vi "script_target_dsf_configuration.vi"(5 "Plugin Timing":T3={"priority"=100, "decimation"=1, "offset"=0}, 7 "configuration version":cluster{"major":u32, "minor":u32, "fix":u32}={"major"=1, "minor"=0, "fix"=0}, 8 "error in":errorcluster, 9 "Target Threads":T1[](array[typedef]), 10 "Target Configuration":T7, 11 "vsd reference":refnum<k24>) -> (0 "error out":errorcluster)   [LabVIEW 2020]
uses:
  NationalInstruments.VeriStand.SystemDefinitionAPI
  controls/target_configuration_cluster.ctl
  <vilib>/addons/VeriStand Custom Device Scripting APIs/Data Sharing Framework/DSF Core.lvlibp/Typedefs/DSF Timing Info.ctl
  controls/thread_configuration_data.ctl
  controls/tx_transfer_group_configuration_data.ctl
  controls/tx_configuration_data.ctl
  controls/rx_transfer_group_configuration_data.ctl
  controls/rx_configuration_data.ctl
  <vilib>/addons/VeriStand Custom Device Scripting APIs/Data Sharing Framework/DSF Core.lvlibp/Typedefs/DSF Engine Plugin Configuration.ctl
  <vilib>/addons/VeriStand Custom Device Scripting APIs/Data Sharing Framework/DSF Core.lvlibp/Typedefs/Core Plugin Configuration.ctl
  <vilib>/addons/VeriStand Custom Device Scripting APIs/Data Sharing Framework/DSF Core.lvlibp/Typedefs/DSF Settings Info.ctl
  <vilib>/addons/VeriStand Custom Device Scripting APIs/Data Sharing Framework/DSF Core.lvlibp/Typedefs/DSF Engine Plugin Thread Configuration.ctl
  <vilib>/addons/VeriStand Custom Device Scripting APIs/Data Sharing Framework/DSF Core.lvlibp/Typedefs/Core Thread Configuration.ctl
  <vilib>/addons/VeriStand Custom Device Scripting APIs/Data Sharing Framework/DSF Core.lvlibp/Typedefs/DSF Engine Transfer Group Configuration.ctl
  <vilib>/addons/VeriStand Custom Device Scripting APIs/Data Sharing Framework/DSF Core.lvlibp/Typedefs/Core Group Configuration.ctl
  <vilib>/addons/VeriStand Custom Device Scripting APIs/Data Sharing Framework/DSF Core.lvlibp/Typedefs/DSF Direction.ctl
  <vilib>/addons/VeriStand Custom Device Scripting APIs/Data Sharing Framework/DSF Core.lvlibp/Typedefs/DSF Timeout Behavior.ctl
  <vilib>/addons/VeriStand Custom Device Scripting APIs/Data Sharing Framework/DSF Core.lvlibp/Typedefs/DSF Engine Transfer Configuration.ctl
  <vilib>/addons/VeriStand Custom Device Scripting APIs/Data Sharing Framework/DSF Core.lvlibp/Typedefs/Core Transfer Configuration.ctl
  <vilib>/addons/VeriStand Custom Device Scripting APIs/Data Sharing Framework/DSF Core.lvlibp/Typedefs/DSF Engine Channel Configuration.ctl
  <vilib>/addons/VeriStand Custom Device Scripting APIs/Data Sharing Framework/DSF Core.lvlibp/Typedefs/Core Channel Configuration.ctl
  <vilib>/addons/VeriStand Custom Device Scripting APIs/Data Sharing Framework/DSF Core.lvlibp/Typedefs/DSF Data Type.ctl
  <vilib>/addons/VeriStand Custom Device Scripting APIs/Data Sharing Framework/DSF Core.lvlibp/Typedefs/DSF Engine Framework Configuration.ctl
  <vilib>/addons/VeriStand Custom Device Scripting APIs/Data Sharing Framework/Data Sharing Framework Custom Device Scripting.lvlib
  <vilib>/addons/VeriStand Custom Device Scripting APIs/Data Sharing Framework/DSF Core.lvlibp
  <vilib>/addons/VeriStand Custom Device Scripting APIs/Data Sharing Framework/DSF Core.lvlibp/Classes/Configuration/Core/Plugin/Plugin Configuration.lvclass
  <vilib>/addons/VeriStand Custom Device Scripting APIs/Data Sharing Framework/DSF Core.lvlibp/Classes/Configuration/Core/Thread/Thread Configuration.lvclass
  <vilib>/addons/VeriStand Custom Device Scripting APIs/Data Sharing Framework/DSF Core.lvlibp/Classes/Configuration/Core/Group/Group Configuration.lvclass
  <vilib>/addons/VeriStand Custom Device Scripting APIs/Data Sharing Framework/DSF Core.lvlibp/Classes/Configuration/Core/Transfer/Transfer Configuration.lvclass
  <vilib>/addons/VeriStand Custom Device Scripting APIs/Data Sharing Framework/DSF Core.lvlibp/Classes/Configuration/Core/Channel/Channel Configuration.lvclass
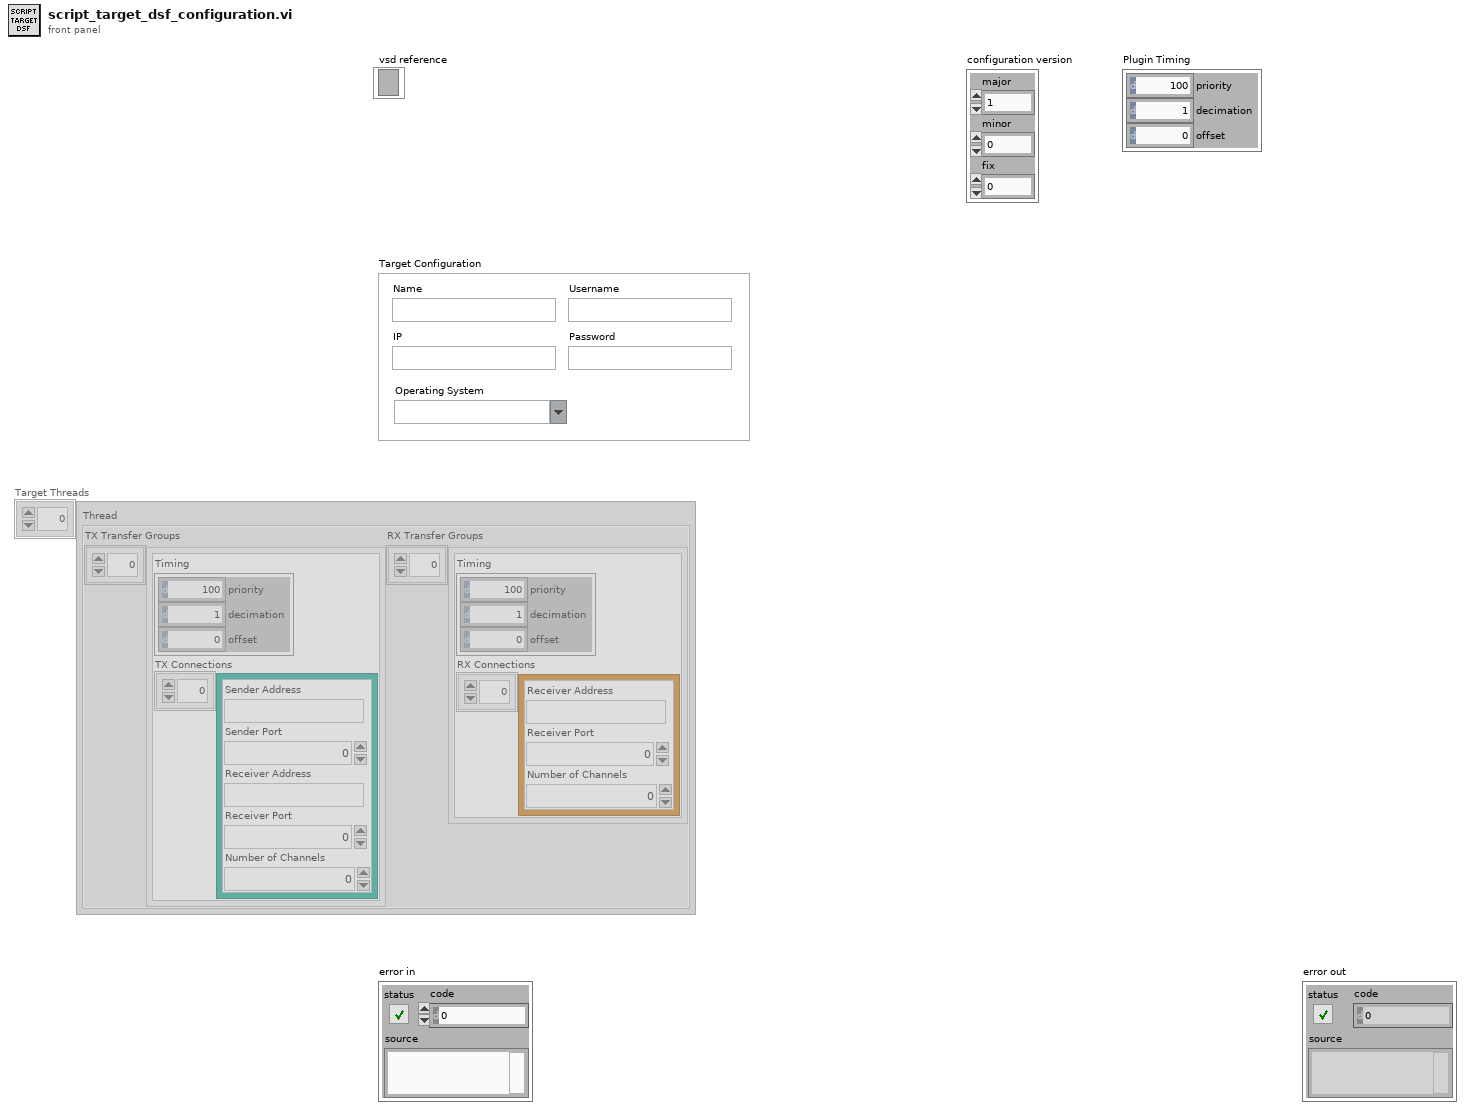
[diagram p1: front panel]
types:
  T1 = typedef "thread_configuration_data.ctl" = cluster{"TX Transfer Groups":T2[], "RX Transfer Groups":T5[]}
  T2 = typedef "tx_transfer_group_configuration_data.ctl" = cluster{"Timing":T3, "TX Connections":T4[]}
  T3 = typedef "DSF Core.lvlibp/DSF Timing Info.ctl" = cluster{"priority":u64, "decimation":u64, "offset":u64}
  T4 = typedef "tx_configuration_data.ctl" = cluster{"Sender Address":string, "Sender Port":u16, "Receiver Address":string, "Receiver Port":u16, "Number of Channels":u16}
  T5 = typedef "rx_transfer_group_configuration_data.ctl" = cluster{"Timing":T3, "RX Connections":T6[]}
  T6 = typedef "rx_configuration_data.ctl" = cluster{"Receiver Address":string, "Receiver Port":u16, "Number of Channels":u16}
  T7 = typedef "target_configuration_cluster.ctl" = cluster{"Name":string, "IP":string, "Username":string, "Password":string, "Operating System":string}
  T8 = typedef "DSF Core.lvlibp/DSF Engine Framework Configuration.ctl" = cluster{"plugins":T9[]}
  T9 = typedef "DSF Core.lvlibp/DSF Engine Plugin Configuration.ctl" = cluster{"core":T10, "component settings":T11[], "threads":T12[]}
  T10 = typedef "DSF Core.lvlibp/Plugin Configuration.lvclass/Core Plugin Configuration.ctl" = cluster{"name":string, "components":string[], "cycle timing":T3}
  T11 = typedef "DSF Core.lvlibp/DSF Settings Info.ctl" = cluster{"component":string, "values":cluster{"key":string, "value":string}[]}
  T12 = typedef "DSF Core.lvlibp/DSF Engine Plugin Thread Configuration.ctl" = cluster{"core":T13, "component settings":T11[], "transfer groups":T14[]}
  T13 = typedef "DSF Core.lvlibp/Thread Configuration.lvclass/Core Thread Configuration.ctl" = cluster{"processor":i32, "priority offset":i16}
  T14 = typedef "DSF Core.lvlibp/DSF Engine Transfer Group Configuration.ctl" = cluster{"core":T15, "component settings":T11[], "transfers":T18[]}
  T15 = typedef "DSF Core.lvlibp/Group Configuration.lvclass/Core Group Configuration.ctl" = cluster{"name":string, "direction":T16, "cycle timing":T3, "timeout behavior":T17, "enable conversion":bool}
  T16 = typedef "DSF Core.lvlibp/DSF Direction.ctl" = enum8{"Tx", "Rx"}
  T17 = typedef "DSF Core.lvlibp/DSF Timeout Behavior.ctl" = enum8{"Increment Late Count", "Throw Error"}
  T18 = typedef "DSF Core.lvlibp/DSF Engine Transfer Configuration.ctl" = cluster{"core":T19, "component settings":T11[], "channels":T20[]}
  T19 = typedef "DSF Core.lvlibp/Transfer Configuration.lvclass/Core Transfer Configuration.ctl" = cluster{"name":string}
  T20 = typedef "DSF Core.lvlibp/DSF Engine Channel Configuration.ctl" = cluster{"core":T21, "component settings":T11[]}
  T21 = typedef "DSF Core.lvlibp/Channel Configuration.lvclass/Core Channel Configuration.ctl" = cluster{"name":string, "units":string, "engine data type":T22, "string data type":T22, "string offset":u64}
  T22 = typedef "DSF Core.lvlibp/DSF Data Type.ctl" = enum8{"Bool", "SGL", "DBL", "I8", "I16", "I32", "I64", "U8", "U16", "U32", "U64"}
  T23 = cluster{"component":string, "values":cluster{"key":string, "value":string}[]}[]
  T24 = typedef "Custom Device API.lvlib/Custom Device Item Ref.ctl" = u64
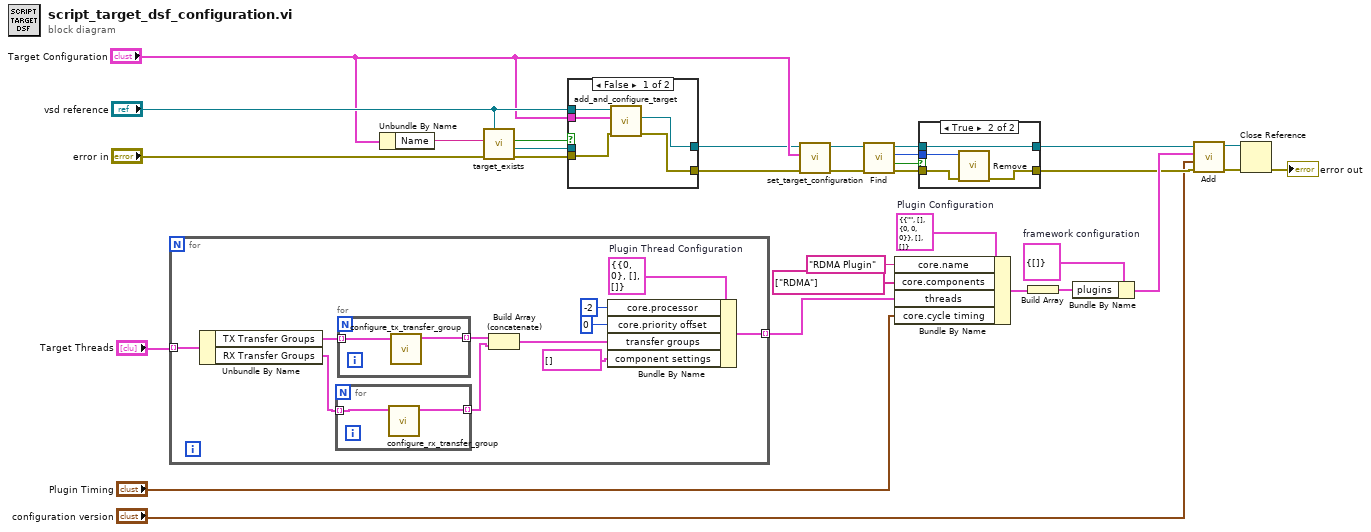
[diagram p0: block diagram]
diagram:
  w25 = T8 {"plugins"=[]}  # framework configuration
  w26 = T9 {"core"={"name"="", "components"=[], "cycle timing"={"priority"=0, "decimation"=0, "offset"=0}}, "component settings"=[], "threads"=[]}  # Plugin Configuration
  n1 = for {
    tunnel: [w37] -> w23 mode=indexing
    tunnel: "Target Threads" -> [w42] mode=indexing
    w40 = T12 {"core"={"processor"=0, "priority offset"=0}, "component settings"=[], "transfer groups"=[]}  # Plugin Thread Configuration
    n2 = Unbundle By Name(w42) -> ("TX Transfer Groups"=w41:T2[], "RX Transfer Groups"=w35:T5[])
    n3 = for {
      tunnel: w35 -> [w45] mode=indexing
      tunnel: [w46] -> w33 mode=indexing
      n4 = call "configure_rx_transfer_group.vi"("RX Transfer Group"=w45) -> ("Transfer Group Configuration"=w46:T14)  [unwired: 10 in]
    }
    n5 = for {
      tunnel: w41 -> [w43] mode=indexing
      tunnel: [w44] -> w34 mode=indexing
      n6 = call "configure_tx_transfer_group.vi"("TX Transfer Group"=w43) -> ("Transfer Group Configuration"=w44:T14)  [unwired: 10 in]
    }
    n7 = Build Array (concatenate)(w34, w33) -> (w32:T14[])
    n8 = Bundle By Name(cluster=w40, "core.processor"=-2, "core.priority offset"=0, "transfer groups"=w32, "component settings"=T23 []) -> (w37:T12)
  }
  n9 = Unbundle By Name("Target Configuration") -> ("Name"=w13:string)
  n10 = call "target_exists.vi"("error in"="error in", "Target Name"=w13, "vsd reference"="vsd reference") -> ("error out"=w9:errorcluster, "target if exists"=w10:refnum<k24>, "Target Exists"=w8:bool)  [unwired: 5 in, 1 out]
  n11 = case shown="False" w8 {
    tunnel: [w51 w53] -> w16
    tunnel: "vsd reference" -> [w50 _]
    tunnel: w10 -> [_ w52]
    tunnel: w9 -> [w49 w53]
    tunnel: "Target Configuration" -> [w48 _]
    tunnel: [w47 w52] -> w6
    frame False {
      n12 = call "add_and_configure_target.vi"("error in"=w49, "Target Configuration"=w48, "vsd reference"=w50) -> ("error out"=w51:errorcluster, "target ref"=w47:refnum<k24>)  [unwired: 6 in, 1 out]
    }
    frame True {
    }
  }
  n13 = call "set_target_configuration.vi"("error in"=w16, "Target Configuration Data"="Target Configuration", "target ref"=w6) -> ("error out"=w14:errorcluster, "target ref out"=w15:refnum<k24>)  [unwired: 7 in]
  n14 = call <vilib>:"Find.vi"("error in"=w14, "target in"=w15) -> ("error out"=w19:errorcluster, "data sharing framework custom device"=w20:T24, "target out"=w5:refnum<k24>, "found?"=w18:bool)  [unwired: 6 in]
  n15 = Bundle By Name(cluster=w26, "core.name"="RDMA Plugin", "core.components"=string[] ["RDMA"], "threads"=w23, "core.cycle timing"="Plugin Timing") -> (w30:T9)
  n16 = case shown="True" w18 {
    tunnel: w20 -> [_ w59]
    tunnel: w19 -> [w55 w58]
    tunnel: [w55 w57] -> w17
    tunnel: w5 -> [w54 w56]
    tunnel: [w54 w56] -> w4
    frame False {
    }
    frame True {
      n17 = call <vilib>:"Remove.vi"("error in"=w58, "data sharing framework custom device"=w59) -> ("error out"=w57:errorcluster)  [unwired: 9 in]
    }
  }
  n18 = Build Array(w30) -> (w29:T9[])
  n19 = Bundle By Name(cluster=w25, "plugins"=w29) -> (w24:T8)
  n20 = call <vilib>:"Add.vi"("error in"=w17, "configuration version"="configuration version", "framework configuration"=w24, "target in"=w4) -> ("error out"=w22:errorcluster, "target out"=w21:refnum<k24>)  [unwired: 5 in, 1 out]
  n21 = Close Reference(reference=w21, error in (no error)=w22) -> (error out=→"error out":errorcluster)
